vi "execute.vi"(8 "error in (no error)":errorcluster, 10 "Context in":refnum<class "Context.lvclass">, 11 "TestForceActuatorCommand in":refnum<class "TestForceActuatorCommand.lvclass">) -> (0 "error out":errorcluster, 2 "Context out":refnum<class "Context.lvclass">, 3 "TestForceActuatorCommand out":refnum<class "TestForceActuatorCommand.lvclass">)   [LabVIEW 2016, in "TestForceActuatorCommand.lvclass"]
uses:
  TestForceActuatorCommand.lvclass
  Context/Context.lvclass
  TestForceActuatorCommand.lvclass/TestForceActuatorCommand.ctl
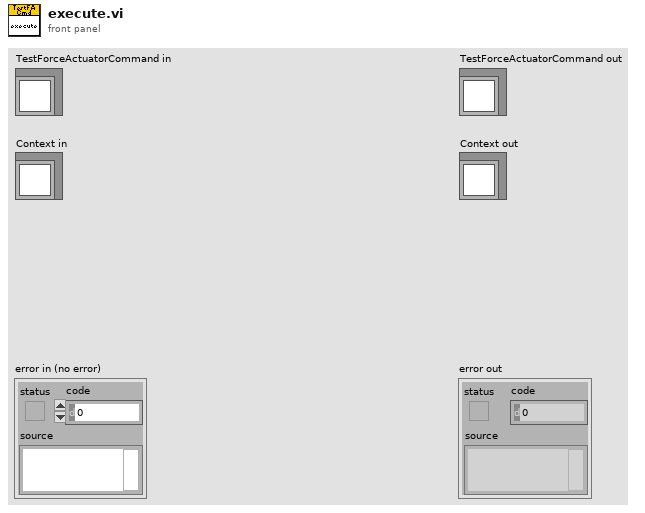
[diagram p1: front panel]
types:
  T1 = typedef "M1M3SupportTopics.lvlib/CommandTestForceActuator.ctl" = cluster{"CommandId":T2, "ActuatorId":i32}
  T2 = typedef "M1M3SupportTopics.lvlib/CommandId.ctl" = i32
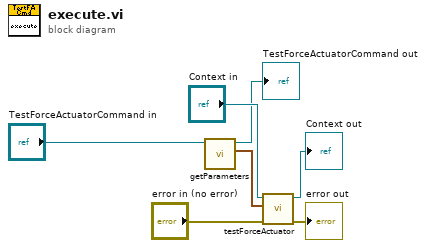
[diagram p0: block diagram]
diagram:
  n1 = call "getParameters.vi"("TestForceActuatorCommand in"="TestForceActuatorCommand in") -> ("Parameters"=w6:T1, "TestForceActuatorCommand out"=→"TestForceActuatorCommand out":refnum<class "TestForceActuatorCommand.lvclass">)  [unwired: 9 in]
  n2 = call-dynamic "testForceActuator.vi"("error in (no error)"="error in (no error)", "Parameters"=w6, "Context in"="Context in") -> ("error out"=→"error out":errorcluster, "Context out"=→"Context out":refnum<class "Context.lvclass">)  [unwired: 7 in]
